vi "Query Memory Catalog.vi"(8 "error in (no error)":errorcluster, 10 "Directory Name":string, 11 "VISA resource name":refnum<visa-resource-name>) -> (0 "error out":errorcluster, 2 "Memory Catalog":string, 3 "VISA resource name out":refnum<visa-resource-name>)   [LabVIEW 2012, in "Keysight B2980 Series.lvlib"]
doc: "Returns the memory usage and availability. Also returns the list of files and folders in the current specified directory."
uses:
  Keysight B2980 Series.lvlib
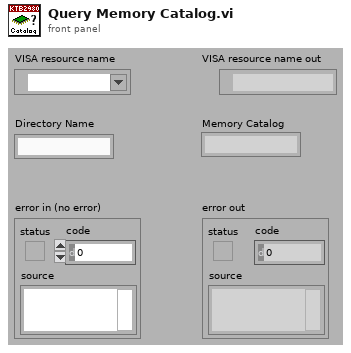
[diagram p1: front panel]
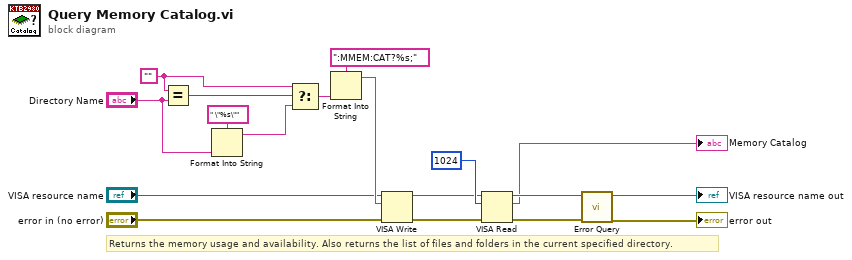
[diagram p0: block diagram]
diagram:
  w5 = ""
  # "Returns the memory usage and availability. Also returns the list of files and folders in the current specified directory."
  n1 = Equal?(x=w5, y="Directory Name") -> (x = y?=w6:bool)
  n2 = Format Into String(format string=" \"%s\"", "Directory Name") -> (resulting string=w1:string)  [unwired: 2 in, 1 out]
  n3 = Select(t=w5, s=w6, f=w1) -> (s? t:f=w4:string)
  n4 = Format Into String(format string=":MMEM:CAT?%s;", w4) -> (resulting string=w17:string)  [unwired: 2 in, 1 out]
  n5 = VISA Write(VISA resource name="VISA resource name", write buffer=w17, error in (no error)="error in (no error)") -> (VISA resource name out=w13:refnum<visa-resource-name>, error out=w12:errorcluster)  [unwired: 1 out]
  n6 = VISA Read(VISA resource name=w13, byte count=u32 1024, error in (no error)=w12) -> (VISA resource name out=w11:refnum<visa-resource-name>, read buffer=→"Memory Catalog":string, error out=w10:errorcluster)  [unwired: 1 out]
  n7 = call "Error Query.vi"("error in (no error)"=w10, "VISA resource name"=w11) -> ("error out"=→"error out":errorcluster, "VISA resource name out"=→"VISA resource name out":refnum<visa-resource-name>)  [unwired: 8 out]
